vi "UpdateGame.vi"(8 "error in (no error)":errorcluster, 10 "Engine in":refnum<class "Engine.lvclass">, 11 "Pong in":refnum<class "Pong.lvclass">) -> (0 "error out":errorcluster, 2 "Engine out":refnum<class "Engine.lvclass">, 3 "Pong out":refnum<class "Pong.lvclass">)   [LabVIEW 2019, in "RT_Game.lvlib" / "Pong.lvclass"]
uses:
  Pong.lvclass
  C:/Users/FreshBob/Dropbox/VIs/myRIO_GameConsole/RT/RT_Game/Game/Game.lvclass
  Engine/Engine.lvclass
  PongPanel/PongPanel.lvclass
  C:/Users/FreshBob/Dropbox/VIs/myRIO_GameConsole/RT/RT_Game/GameObject/GameObject.lvclass
  C:/Users/FreshBob/Dropbox/VIs/myRIO_GameConsole/RT/RT_Game/RT_Sprite/RT_Sprite.lvclass
  PongBall/PongBall.lvclass
  Menu/States.ctl
  Game/Game.lvclass/Game.ctl
  Pong.lvclass/Pong.ctl
  TileTime/TileTimer.lvclass/TileTimer.ctl
  Game/Write Sprite3.vi
  Game/Read Sprite1.vi
  Game/Read Sprite2.vi
  Game/Read Sprite3.vi
  Game/Read State.vi
  TileTime/Write Count.vi
  Game/Write Sprite1.vi
  Game/Write Sprite2.vi
  Engine/Globals.vi
  RT_Sprite/RT_Sprite.lvclass
  TileTime/TileTimer.lvclass
  GameObject/GameObject.lvclass
  Game/Game.lvclass
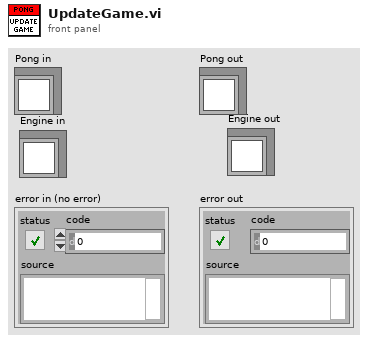
[diagram p1: front panel]
types:
  T1 = typedef "RT_Game.lvlib/Game.lvclass/States.ctl" = enum16{"Init", "Restart", "Menu", "Game", "Resume", "ToggleSingleplayer", "LoadNextGame", "ExitToMenu", "NewHighscore", "GameOver", "SlideOut", "FadeToMenu", "StartFadeToMenu"}
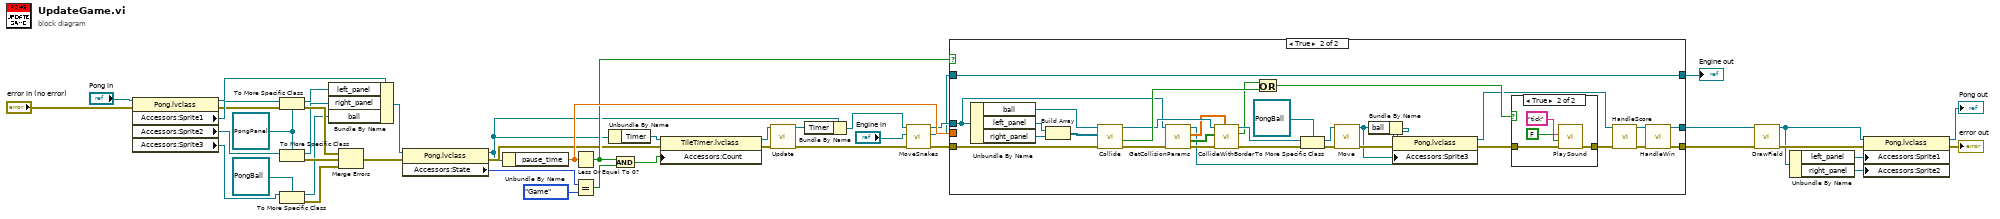
[diagram p0: block diagram]
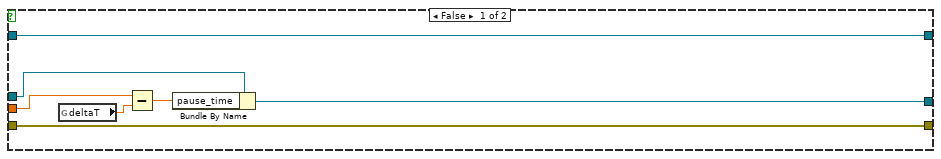
[diagram p2: hidden frame]
diagram:
  w42 = refnum<class "PongPanel.lvclass"> refnum ("RT_Game.lvlib:PongPanel.lvclass")
  n1 = property class="Pong.lvclass"(reference="Pong in", error in="error in (no error)") -> (reference out=w26:refnum<class "Pong.lvclass">, error out=w33:errorcluster, "Accessors:Sprite1"=w36:refnum<class "RT_Sprite.lvclass">, "Accessors:Sprite2"=w37:refnum<class "RT_Sprite.lvclass">, "Accessors:Sprite3"=w41:refnum<class "RT_Sprite.lvclass">)
  n2 = To More Specific Class(target class=w42, reference=w36, error in=w33) -> (specific class reference=w24:refnum<class "PongPanel.lvclass">, error out=w35:errorcluster)
  n3 = To More Specific Class(target class=w42, reference=w37) -> (specific class reference=w23:refnum<class "PongPanel.lvclass">, error out=w39:errorcluster)  [unwired: 1 in]
  n4 = To More Specific Class(target class=refnum<class "PongBall.lvclass"> refnum ("RT_Game.lvlib:PongBall.lvclass"), reference=w41) -> (specific class reference=w22:refnum<class "PongBall.lvclass">, error out=w40:errorcluster)  [unwired: 1 in]
  n5 = Bundle By Name(cluster=w26, "left_panel"=w24, "right_panel"=w23, "ball"=w22) -> (w14:refnum<class "Pong.lvclass">)
  n6 = Merge Errors(w35, w39, w40) -> (w38:errorcluster)
  n7 = property class="Pong.lvclass"(reference=w14, error in=w38) -> (reference out=w13:refnum<class "Pong.lvclass">, error out=w15:errorcluster, "Accessors:State"=w12:T1)
  n8 = Unbundle By Name(w13) -> ("pause_time"=w31:dbl)
  n9 = Less Or Equal To 0?(x=w31) -> (x <= 0?=w16:bool)
  n10 = Equal?(x=w12, y=States."Game") -> (x = y?=w9:bool)
  n11 = Unbundle By Name(w13) -> ("Timer"=w18:refnum<class "TileTimer.lvclass">)
  n12 = And(x=w16, y=w9) -> (x .and. y?=w10:bool)
  n13 = property class="TileTimer.lvclass"(reference=w18, error in=w15, "Accessors:Count"=w10) -> (reference out=w17:refnum<class "TileTimer.lvclass">, error out=w19:errorcluster)
  n14 = call-dynamic "Update.vi"("error in (no error)"=w19, "TileTimer in"=w17) -> ("error out"=w21:errorcluster, "TileTimer out"=w20:refnum<class "TileTimer.lvclass">)  [unwired: 8 in]
  n15 = Bundle By Name(cluster=w13, "Timer"=w20) -> (w8:refnum<class "Pong.lvclass">)
  n16 = call-dynamic "MoveSnakes.vi"("error in (no error)"=w21, "Engine in"="Engine in", "Pong in"=w8) -> ("error out"=w29:errorcluster, "Engine out"=w1:refnum<class "Engine.lvclass">, "Pong out"=w5:refnum<class "Pong.lvclass">)  [unwired: 6 in]
  n17 = case shown="True" w16 {
    tunnel: w5 -> [w46 w58]
    tunnel: w29 -> [w51 w81]
    tunnel: [w50 w65] -> w25
    tunnel: [w51 w67] -> w30
    tunnel: w31 -> [w49 _]
    tunnel: [w45 w61] -> w6
    tunnel: w1 -> [w45 w61]
    frame False {
      n18 = global read "Globals.vi" "deltaT"() -> (w48:dbl)
      n19 = Subtract(x=w49, y=w48) -> (x-y=w47:dbl)
      n20 = Bundle By Name(cluster=w46, "pause_time"=w47) -> (w50:refnum<class "Pong.lvclass">)
    }
    frame True {
      n21 = Unbundle By Name(w58) -> ("ball"=w57:refnum<class "PongBall.lvclass">, "left_panel"=w59:refnum<class "PongPanel.lvclass">, "right_panel"=w60:refnum<class "PongPanel.lvclass">)
      n22 = Build Array(w59, w60) -> (w56:refnum<class "PongPanel.lvclass">[])
      n23 = call "Collide.vi"("error in (no error)"=w81, "ColliderObjects in"=w56, "Object in"=w57) -> ("error out"=w82:errorcluster, "collided"=w79:bool, "Object out"=w74:refnum<class "GameObject.lvclass">)  [unwired: 5 in, 1 out]
      n24 = call-dynamic "GetCollisionParams.vi"("error in (no error)"=w82, "Pong in"=w58) -> ("error out"=w63:errorcluster, "UpDownLeftRightCollide"=w72:bool[], "UpDownLeftRightBounce"=w64:dbl[], "Pong out"=w62:refnum<class "Pong.lvclass">)  [unwired: 6 in]
      n25 = call "CollideWithBorder.vi"("UpDownLeftRightBounce"=w64, "error in (no error)"=w63, "UpDownLeftRightCollide"=w72, "Object in"=w74) -> ("error out"=w75:errorcluster, "collided?"=w70:bool, "Object out"=w73:refnum<class "GameObject.lvclass">)  [unwired: 5 in]
      n26 = Or(x=w70, y=w79) -> (x .or. y?=w71:bool)
      n27 = To More Specific Class(target class=refnum<class "PongBall.lvclass"> refnum ("PongBall in"), reference=w73, error in=w75) -> (specific class reference=w76:refnum<class "PongBall.lvclass">, error out=w78:errorcluster)
      n28 = call "Move.vi"("error in (no error)"=w78, "PongBall in"=w76) -> ("error out"=w80:errorcluster, "PongBall out"=w52:refnum<class "PongBall.lvclass">)  [unwired: 8 in]
      n29 = Bundle By Name(cluster=w62, "ball"=w52) -> (w54:refnum<class "Pong.lvclass">)
      n30 = property class="Pong.lvclass"(reference=w54, error in=w80, "Accessors:Sprite3"=w52) -> (reference out=w53:refnum<class "Pong.lvclass">, error out=w55:errorcluster)
      n31 = case shown="True" w71 {
        tunnel: w55 -> [w83 w87]
        tunnel: [w83 w86] -> w69
        frame False {
        }
        frame True {
          n32 = call "PlaySound.vi"("error in (no error)"=w87, "Overwrite"=FALSE, "Name"="tick") -> ("error out"=w86:errorcluster)  [unwired: 8 in]
        }
      }
      n33 = call "HandleScore.vi"("error in (no error)"=w69, "Pong in"=w53) -> ("error out"=w68:errorcluster, "Pong out"=w66:refnum<class "Pong.lvclass">)  [unwired: 8 in]
      n34 = call "HandleWin.vi"("error in (no error)"=w68, "Pong in"=w66) -> ("error out"=w67:errorcluster, "Pong out"=w65:refnum<class "Pong.lvclass">)  [unwired: 8 in]
    }
  }
  "Engine out" <- w6
  n35 = call "DrawField.vi"("error in (no error)"=w30, "Pong in"=w25) -> ("error out"=w32:errorcluster, "Pong out"=w4:refnum<class "Pong.lvclass">)  [unwired: 8 in]
  n36 = Unbundle By Name(w4) -> ("left_panel"=w3:refnum<class "PongPanel.lvclass">, "right_panel"=w2:refnum<class "PongPanel.lvclass">)
  n37 = property class="Pong.lvclass"(reference=w4, error in=w32, "Accessors:Sprite1"=w3, "Accessors:Sprite2"=w2) -> (reference out=→"Pong out":refnum<class "Pong.lvclass">, error out=→"error out":errorcluster)
